vi "Tooltip and Description Message.vi"() -> ()   [LabVIEW 2021, in "myRIOMetaDataObj.lvclass"]
uses:
  myRIOMetaDataObj.lvclass
panel:
  in  "FPGA Selector Tooltip":string="Lists FPGA personalities."
  in  "FPGA Selector Description":string="Lists FPGA personalities. Different FPGA personalities enable you to use different %s VIs."
  in  "IP Tooltip":string="Specifies the IP address or hostname of the %s target."
  in  "IP Description":string="Specifies the IP address or hostname of the %s target."
  in  "Target List Tooltip":string="Lists %s targets determined by the Target."
  in  "Target List Description":string="Lists %s targets determined by the <b>Target</b>."
  in  "Target Tooltip":string="Specifies the categories of %s targets."
  in  "Target Description":string="Specifies the categories of %s targets. You can specify %s %s target that is connected to the host computer with a USB cable or over a wireless network. You can also specify a generic %s target, or specify a %s target with an IP address or hostname."
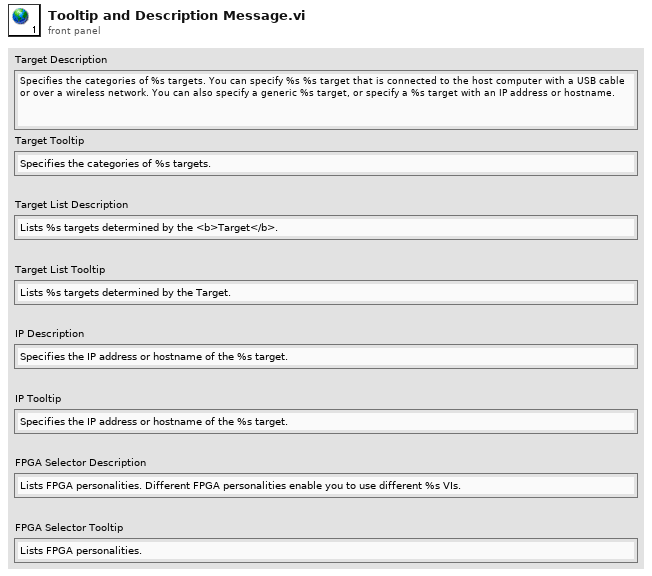
[diagram p1: front panel]
diagram:
